vi "Subscribe.vi"(8 "error in (no error)":errorcluster, 10 "Subscription Request":refnum<class "SubscriptionRequest.lvclass">, 11 "MonitoredMediator In":refnum<class "MonitoredMediator.lvclass">) -> (0 "error out":errorcluster, 3 "MonitoredMediator Out":refnum<class "MonitoredMediator.lvclass">)   [LabVIEW 2018, in "MVA Framework.lvlib" / "MonitoredMediator.lvlib" / "MonitoredMediator.lvclass"]
doc: "订阅"
uses:
  MonitoredMediator.lvclass
  IMediator/SubscriptionRequest/SubscriptionRequest.lvclass
  MonitoredMediator.lvclass/MonitoredMediator.ctl
  IBusMonitor/IBusMonitor.lvclass
  Mediator/Mediator/Mediator.lvclass
panel:
  # "What does subscriber want? (Datum Name and Type)\nHow does it get sent? (Transport)\nUnder what conditions? (SubscriptionPolicy)"
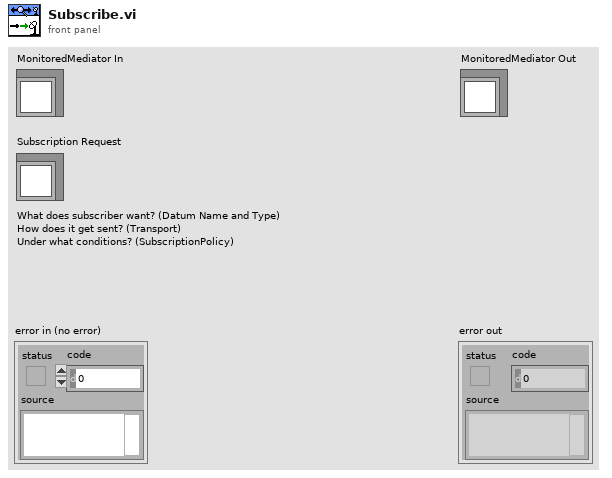
[diagram p1: front panel]
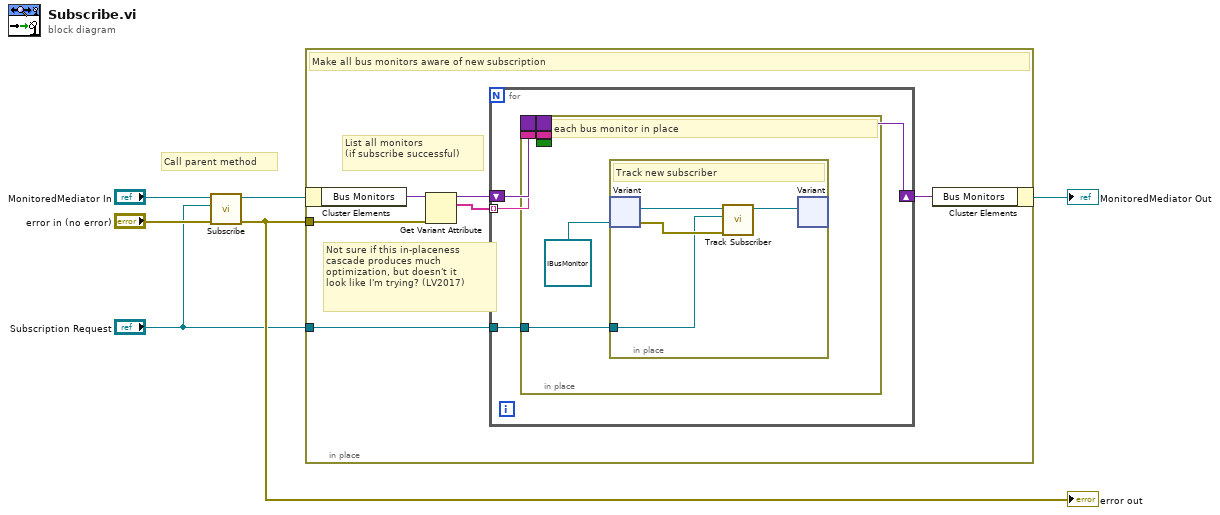
[diagram p0: block diagram]
diagram:
  # "Call parent method"
  n1 = call-parent "Subscribe.vi"("error in (no error)"="error in (no error)", "Subscription Request"="Subscription Request", "Mediator In"="MonitoredMediator In") -> ("error out"=w2:errorcluster, "Mediator Out"=w4:refnum<class "MonitoredMediator.lvclass">)  [unwired: 7 in]
  "error out" <- w2
  n2 = in-place {
    in-place-border: w2 -> [w8]
    in-place-border: "Subscription Request" -> [w7]
    # "Not sure if this in-placeness\ncascade produces much\noptimization, but doesn't it\nlook like I'm trying? (LV2017)"
    # "List all monitors\n(if subscribe successful)"
    # "Make all bus monitors aware of new subscription"
    n3 = in-place-cluster #1(w4) -> ("Bus Monitors"=w11:variant)
    n4 = Get Variant Attribute(Variant=w11, error in=w8) -> (duplicate Variant=w10:variant, names=w9:string[])  [unwired: 2 in, 2 out]
    n5 = for {
      tunnel: w9 -> [w14] mode=indexing
      shift-right: [w16] -> w12
      shift-left: w10 -> [w15]
      tunnel: w7 -> [w13]
      n6 = in-place {
        border: w15 -> [_]
        border: w14 -> [_]
        border: [_] -> w16
        border: _ -> [_]
        border: _ -> [_]
        in-place-border: w13 -> [w17]
        # "Read each bus monitor in place"
        n7 = in-place {
          in-place-border: w17 -> [w21]
          # "Track new subscriber"
          n8 = in-place-variant #2(w20, refnum<class "IBusMonitor.lvclass"> refnum ("IBusMonitor")) -> (w24:refnum<class "IBusMonitor.lvclass">, w22:errorcluster)
          n9 = call-dynamic "Track Subscriber.vi"("error in (no error)"=w22, "SubscriptionRequest"=w21, "IBusMonitor In"=w24) -> ("IBusMonitor Out"=w23:refnum<class "IBusMonitor.lvclass">)  [unwired: 7 in, 1 out]
          n10 = in-place-variant #2(w23) -> (w19:variant)  [unwired: 1 out]
        }
      }
    }
    n11 = in-place-cluster #1("Bus Monitors"=w12) -> (→"MonitoredMediator Out":refnum<class "MonitoredMediator.lvclass">)
  }
